vi "FTW-Actor-CreateSelfRef.vi"(0 "FTW Actor":refnum<class "FTW-Actor.lvclass">, 11 "error in":errorcluster) -> (4 "FTW Actor out":refnum<class "FTW-Actor.lvclass">, 6 "Reference to Self":refnum<class "FTW-ActorReference.lvclass">, 15 "error out":errorcluster)   [LabVIEW 2014, in "FTW-Actor.lvclass"]
uses:
  FTW-Actor.lvclass
  Reference/FTW-ActorReference.lvclass
panel:
  # "Inputs"
  # "Outputs"
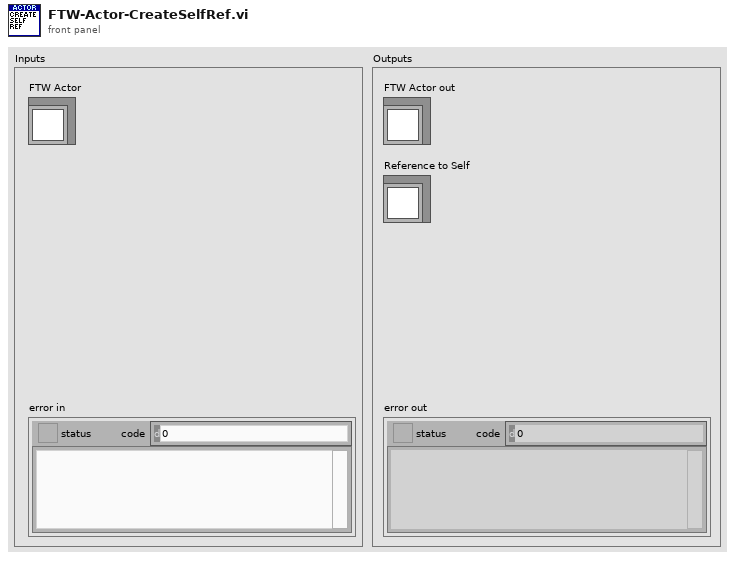
[diagram p1: front panel]
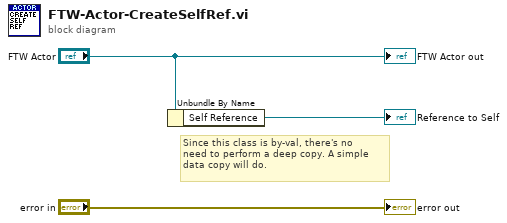
[diagram p0: block diagram]
diagram:
  # "Since this class is by-val, there's no\nneed to perform a deep copy. A simple\ndata copy will do."
  n1 = Unbundle By Name("FTW Actor") -> ("Self Reference"=→"Reference to Self":refnum<class "FTW-ActorReference.lvclass">)
  "error out" <- "error in"
  "FTW Actor out" <- "FTW Actor"
